vi "Convert Channel Values to PWM Measure Digital Settings.vi"(9 "Length":i32, 10 "Index":i32, 11 "Channel Values in":dbl[](array[numeric])) -> (2 "PWM Measure Digital Settings":T1, 3 "Channel Values out":dbl[](array[numeric]))   [LabVIEW 2018, in "FPGA Addon Engine.lvlib"]
uses:
  FPGA Addon Engine.lvlib
  Submodules/Source/Types/PWM.Measure.Digital.Settings.ctl
  Submodules/Source/Speciality FPGA IO.lvlib
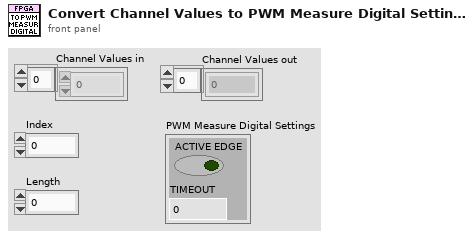
[diagram p1: front panel]
types:
  T1 = typedef "Speciality FPGA IO.lvlib/PWM.Measure.Digital.Settings.ctl" = cluster{"ACTIVE EDGE":bool, "TIMEOUT":u32}
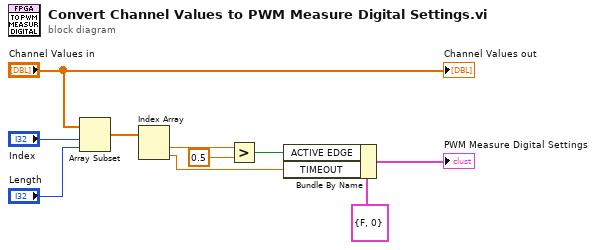
[diagram p0: block diagram]
diagram:
  n1 = Array Subset(array="Channel Values in", index="Index", length="Length") -> (w1:dbl[])
  n2 = Index Array(array=w1) -> (element #1=w4:dbl, element #2=w5:dbl)  [unwired: 2 in]
  n3 = Greater?(x=w4, y=0.5) -> (0:w2:bool)
  n4 = Bundle By Name(cluster=T1 {"ACTIVE EDGE"=FALSE, "TIMEOUT"=0}, "ACTIVE EDGE"=w2, "TIMEOUT"=w5) -> (→"PWM Measure Digital Settings":T1)
  "Channel Values out" <- "Channel Values in"
